vi "Untitled 1.vi"() -> ()   [LabVIEW 2023]
uses:
  Control Timer.ctl
panel:
  out "Mixing":bool
  out "Boiling milk":bool
  out "Adding Milk":bool
  out "Boiling":bool
  out "Adding Coffee":bool
  out "Adding Water":bool
  in  "WHITE COFFEE":bool
  in  "CAPUCCINO":bool
  in  "ESPRESSO LONG":bool
  in  "ESPRESSO SHORT":bool
  in  "STOP":bool
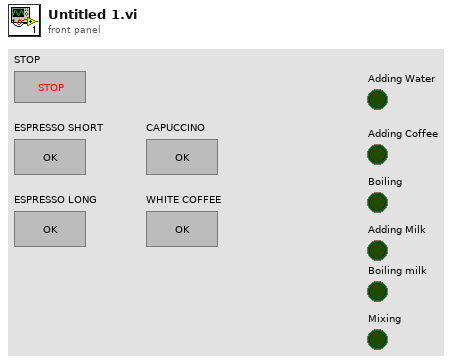
[diagram p1: front panel]
types:
  T1 = typedef "Control Timer.ctl" = enum16{"Timecheck", "Reset"}
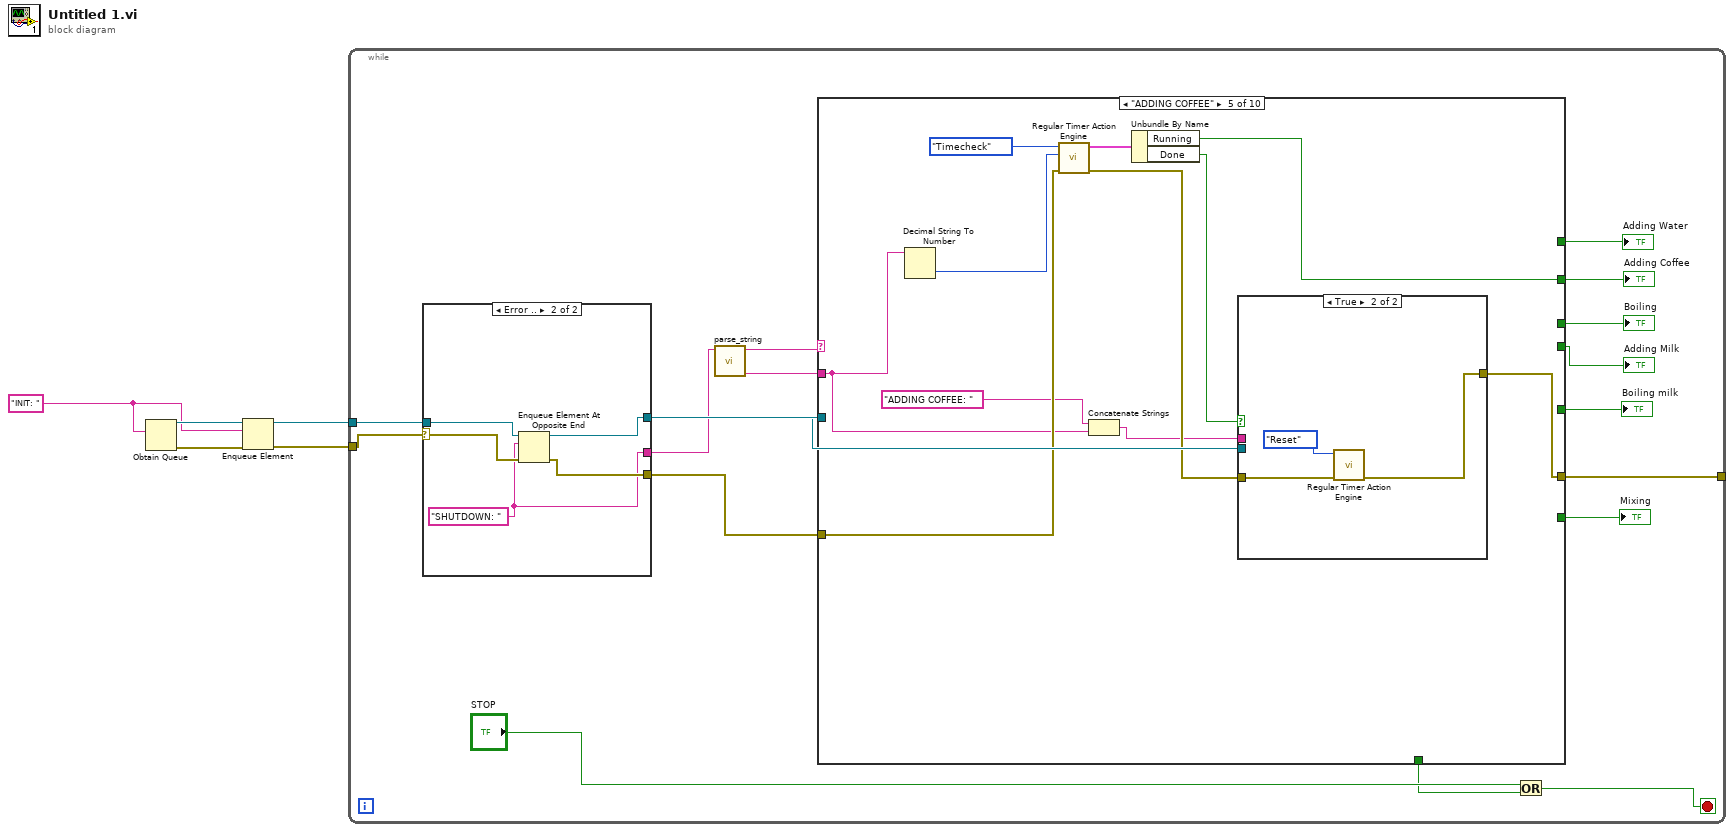
[diagram p0: block diagram]
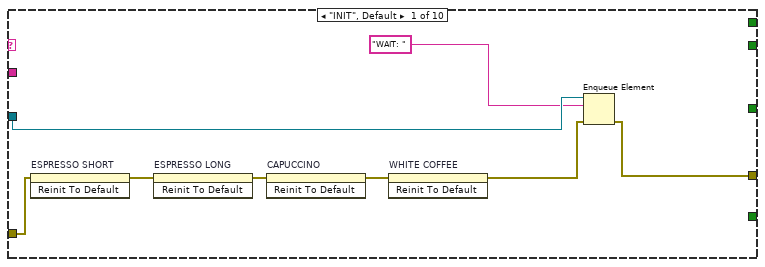
[diagram p2: hidden frame]
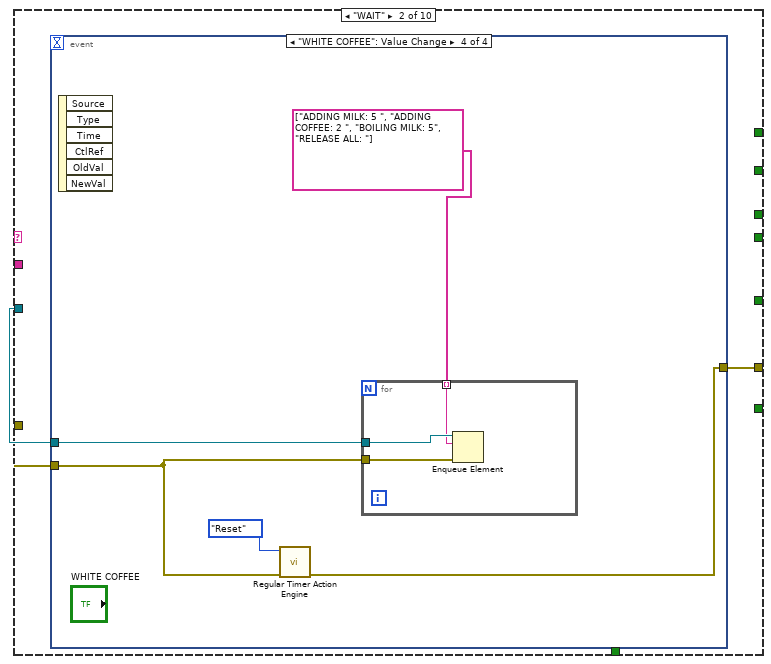
[diagram p3: hidden frame]
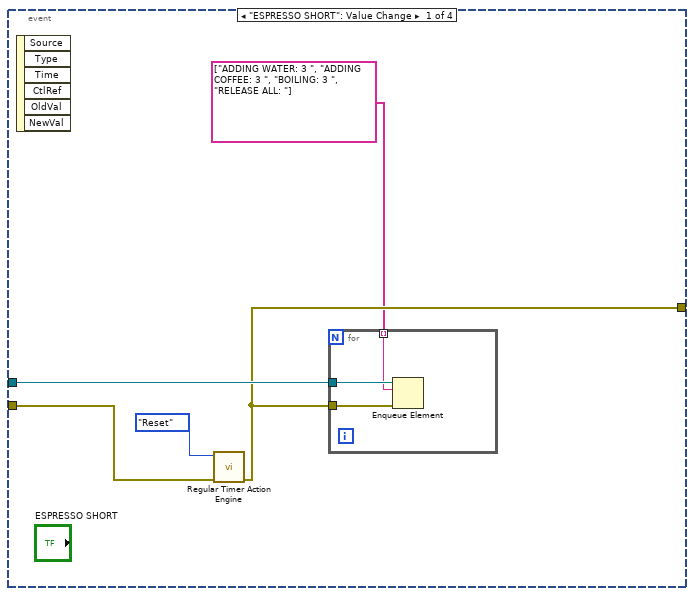
[diagram p4: hidden frame]
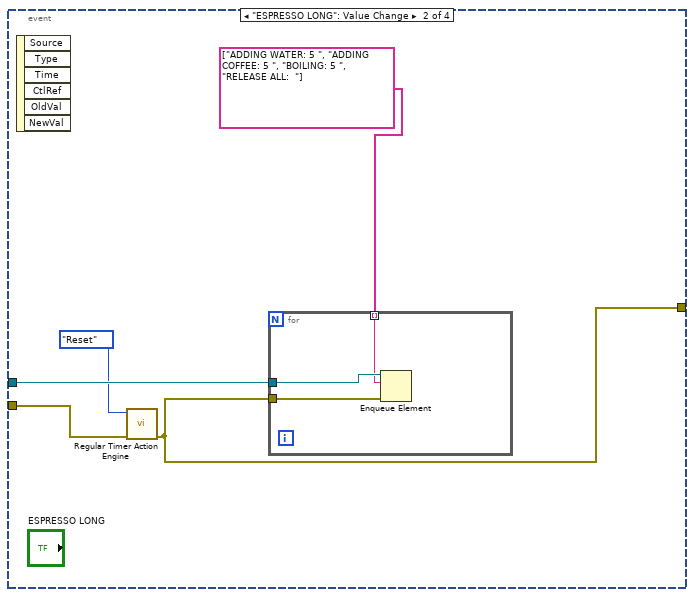
[diagram p5: hidden frame]
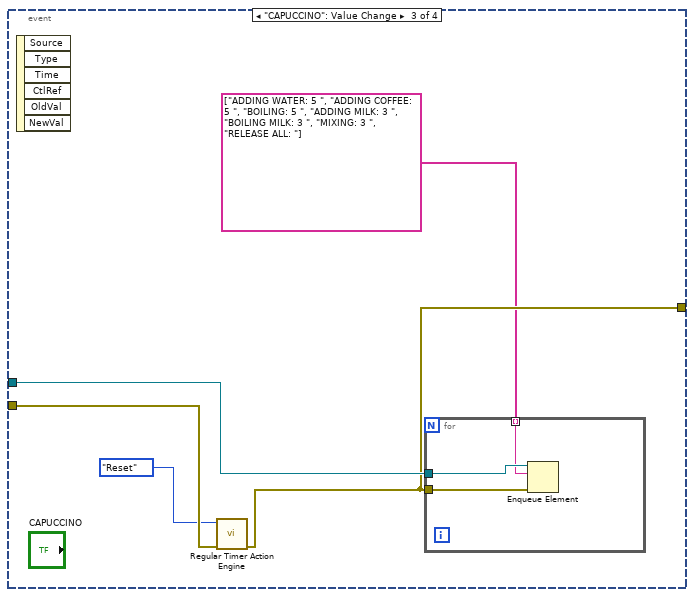
[diagram p6: hidden frame]
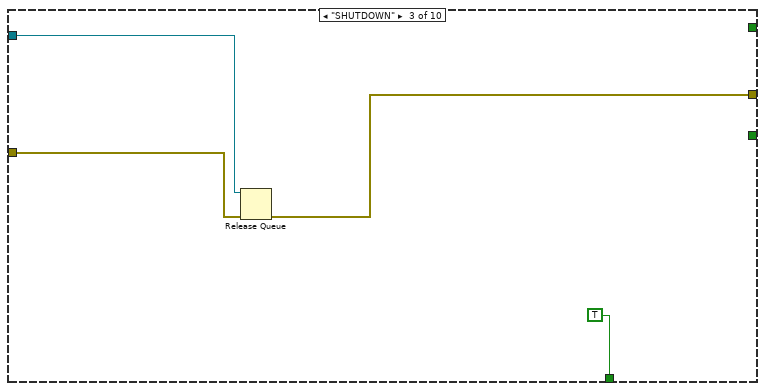
[diagram p7: hidden frame]
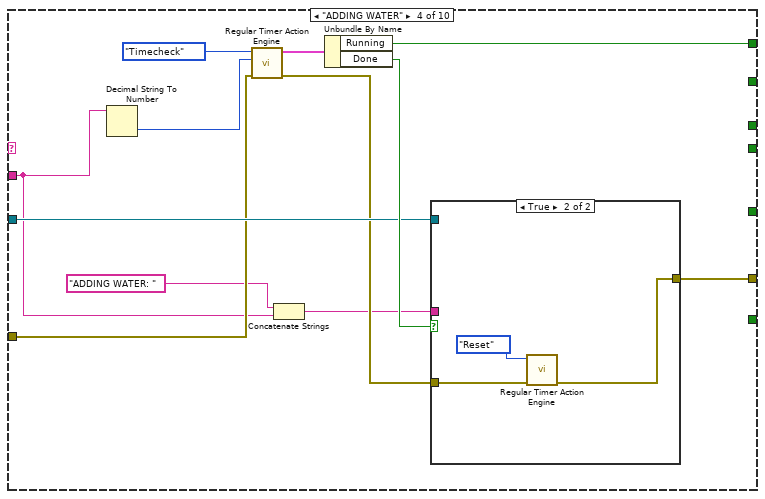
[diagram p8: hidden frame]
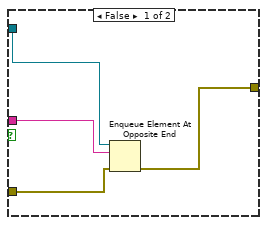
[diagram p9: hidden frame]
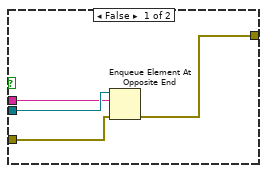
[diagram p10: hidden frame]
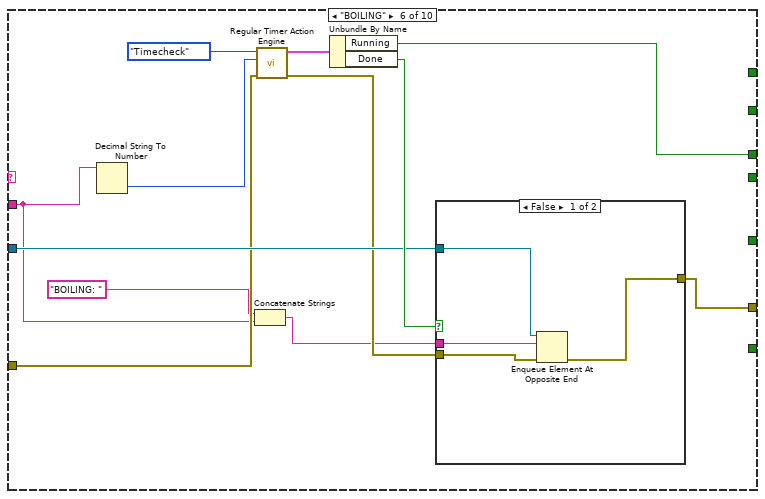
[diagram p11: hidden frame]
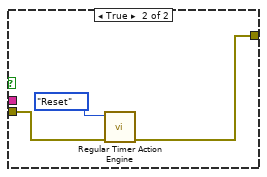
[diagram p12: hidden frame]
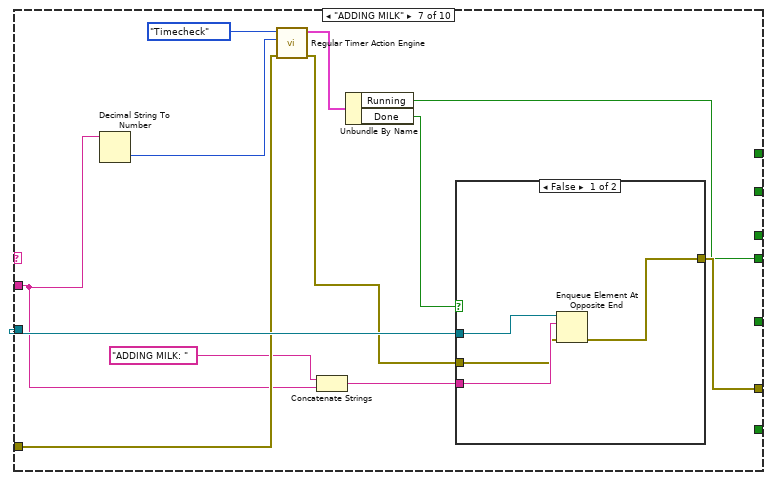
[diagram p13: hidden frame]
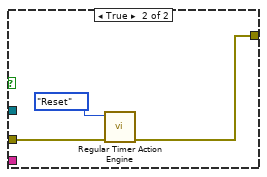
[diagram p14: hidden frame]
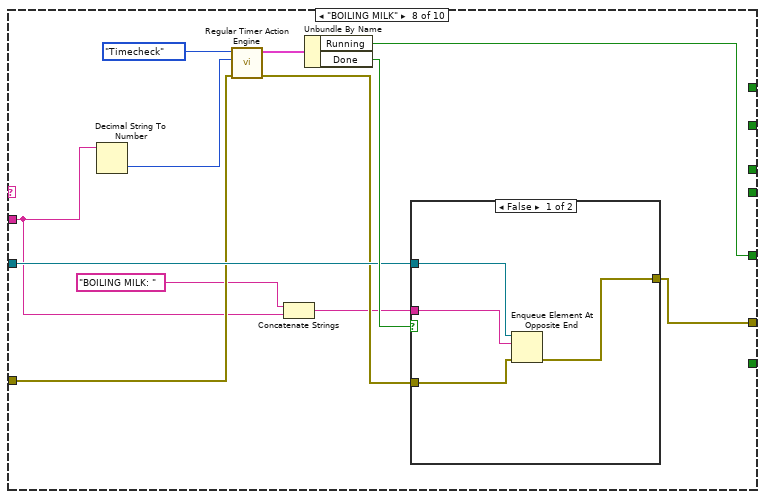
[diagram p15: hidden frame]
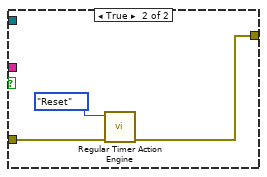
[diagram p16: hidden frame]
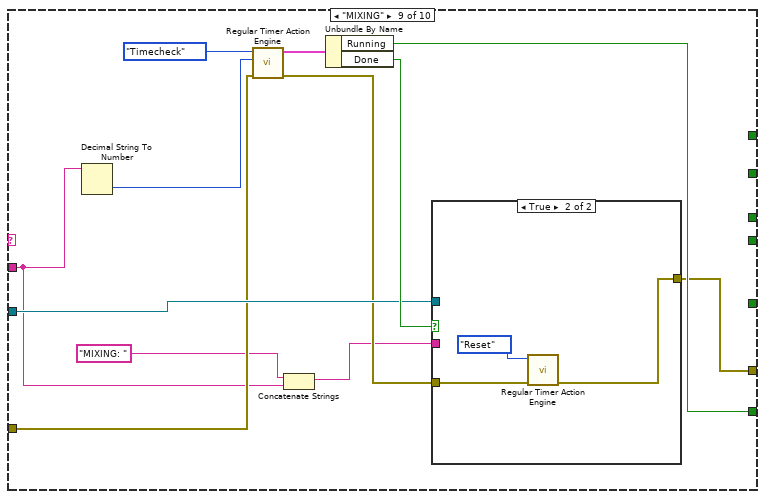
[diagram p17: hidden frame]
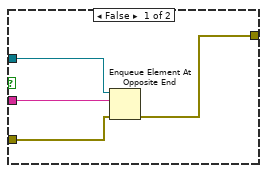
[diagram p18: hidden frame]
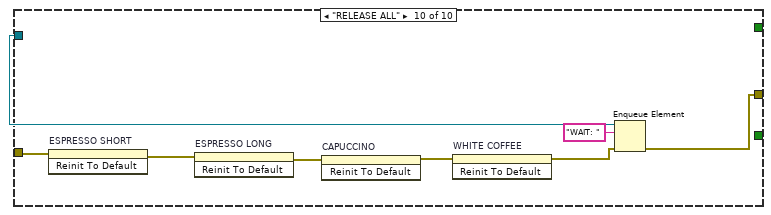
[diagram p19: hidden frame]
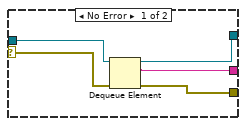
[diagram p20: hidden frame]
diagram:
  w1 = "INIT: "
  n1 = Obtain Queue(element data type=w1) -> (queue out=w5:refnum<queue>, error out=w4:errorcluster)  [unwired: 4 in, 1 out]
  n2 = Enqueue Element(queue=w5, element=w1, error in (no error)=w4) -> (queue out=w2:refnum<queue>, error out=w3:errorcluster)  [unwired: 1 in, 1 out]
  n3 = while {
    tunnel: w3 -> [w22]
    tunnel: w2 -> [w21]
    tunnel: [w18] -> _
    stop <- w9 stop-if-true
    n4 = case shown="Error .." w22 {
      selector: w22 -> [w196 w201]
      tunnel: w21 -> [w195 w199]
      tunnel: [w194 w198] -> w19
      tunnel: [w193 w200] -> w20
      tunnel: [w192 w197] -> w6
      frame No Error {
        n5 = Dequeue Element(queue=w195, error in (no error)=w196) -> (queue out=w194:refnum<queue>, element=w192:string, error out=w193:errorcluster)  [unwired: 1 in, 1 out]
      }
      frame Error {
        w197 = "SHUTDOWN: "
        n6 = Enqueue Element At Opposite End(queue=w199, element=w197, error in (no error)=w201) -> (queue out=w198:refnum<queue>, error out=w200:errorcluster)  [unwired: 1 in, 1 out]
      }
    }
    n7 = call "parse_string.vi"("Input"=w6) -> ("Argument"=w7:string, "State"=w8:string)  [unwired: 9 in]
    n8 = case shown="\"ADDING COFFEE\"" w8 {
      tunnel: w20 -> [w24 w32 w69 w75 w94 w113 w132 w151 w169 w191]
      tunnel: w19 -> [w30 w33 w68 w76 w97 w116 w134 w154 w172 w186]
      tunnel: [w25 w31 w66 w77 w95 w114 w135 w152 w170 w185] -> w18
      tunnel: [_ _ _ w79 _ _ _ _ _ _] -> w17
      tunnel: [_ _ _ _ w96 _ _ _ _ _] -> w16
      tunnel: [_ _ _ _ _ w115 _ _ _ _] -> w15
      tunnel: [_ _ _ _ _ _ w133 _ _ _] -> w14
      tunnel: [_ _ _ _ _ _ _ w153 _ _] -> w13
      tunnel: [_ _ _ _ _ _ _ _ w171 _] -> w12
      tunnel: [_ _ TRUE _ _ _ _ _ _ _] -> w10
      tunnel: w7 -> [_ _ _ w70 w89 w108 w127 w146 w165 _]
      frame "INIT", Default {
        n9 = invoke on="ESPRESSO SHORT" class="Bool" method="Reinit To Default"(error in=w24) -> (error out=w29:errorcluster)  [unwired: 2 in, 2 out]
        n10 = invoke on="ESPRESSO LONG" class="Bool" method="Reinit To Default"(error in=w29) -> (error out=w28:errorcluster)  [unwired: 2 in, 2 out]
        n11 = invoke on="CAPUCCINO" class="Bool" method="Reinit To Default"(error in=w28) -> (error out=w27:errorcluster)  [unwired: 2 in, 2 out]
        n12 = invoke on="WHITE COFFEE" class="Bool" method="Reinit To Default"(error in=w27) -> (error out=w26:errorcluster)  [unwired: 2 in, 2 out]
        n13 = Enqueue Element(queue=w30, element="WAIT: ", error in (no error)=w26) -> (error out=w25:errorcluster)  [unwired: 1 in, 2 out]
      }
      frame "WAIT" {
        n14 = event shown="[3] \"WHITE COFFEE\": Value Change" {
          selector: _ -> [_ _ _ _]
          dyn-events: _ -> [_ _ _ _]
          timeout: _ -> [_ _ _ _]
          tunnel: w33 -> [w38 w46 w54 w62]
          tunnel: w32 -> [w36 w44 w53 w59]
          tunnel: [w35 w43 w51 w60] -> w31
          event "ESPRESSO SHORT": Value Change {
            n15 = event-data() -> ()  [unwired: 1 in, 6 out]
            n16 = call "Regular Timer Action Engine.vi"("Enum"=Control_Timer."Reset", "error in"=w36) -> ("error out"=w35:errorcluster)  [unwired: 7 in, 1 out]
            n17 = for {
              tunnel: w38 -> [w41]
              tunnel: w35 -> [w40]
              tunnel: string[] ["ADDING WATER: 3 ", "ADDING COFFEE: 3 ", "BOILING: 3 ", "RELEASE ALL: "] -> [w39] mode=indexing
              n18 = Enqueue Element(queue=w41, element=w39, error in (no error)=w40) -> ()  [unwired: 1 in, 3 out]
            }
          }
          event "ESPRESSO LONG": Value Change {
            n19 = event-data() -> ()  [unwired: 1 in, 6 out]
            n20 = call "Regular Timer Action Engine.vi"("Enum"=Control_Timer."Reset", "error in"=w44) -> ("error out"=w43:errorcluster)  [unwired: 7 in, 1 out]
            n21 = for {
              tunnel: w46 -> [w49]
              tunnel: w43 -> [w48]
              tunnel: string[] ["ADDING WATER: 5 ", "ADDING COFFEE: 5 ", "BOILING: 5 ", "RELEASE ALL:  "] -> [w47] mode=indexing
              n22 = Enqueue Element(queue=w49, element=w47, error in (no error)=w48) -> ()  [unwired: 1 in, 3 out]
            }
          }
          event "CAPUCCINO": Value Change {
            n23 = event-data() -> ()  [unwired: 1 in, 6 out]
            n24 = call "Regular Timer Action Engine.vi"("Enum"=Control_Timer."Reset", "error in"=w53) -> ("error out"=w51:errorcluster)  [unwired: 7 in, 1 out]
            n25 = for {
              tunnel: w54 -> [w57]
              tunnel: w51 -> [w56]
              tunnel: string[] ["ADDING WATER: 5 ", "ADDING COFFEE: 5 ", "BOILING: 5 ", "ADDING MILK: 3 ", "BOILING MILK: 3 ", "MIXING: 3 ", "RELEASE ALL: "] -> [w55] mode=indexing
              n26 = Enqueue Element(queue=w57, element=w55, error in (no error)=w56) -> ()  [unwired: 1 in, 3 out]
            }
          }
          event "WHITE COFFEE": Value Change {
            n27 = event-data() -> ()  [unwired: 1 in, 6 out]
            n28 = call "Regular Timer Action Engine.vi"("Enum"=Control_Timer."Reset", "error in"=w59) -> ("error out"=w60:errorcluster)  [unwired: 7 in, 1 out]
            n29 = for {
              tunnel: w62 -> [w65]
              tunnel: w59 -> [w64]
              tunnel: string[] ["ADDING MILK: 5 ", "ADDING COFFEE: 2 ", "BOILING MILK: 5", "RELEASE ALL: "] -> [w63] mode=indexing
              n30 = Enqueue Element(queue=w65, element=w63, error in (no error)=w64) -> ()  [unwired: 1 in, 3 out]
            }
          }
        }
      }
      frame "SHUTDOWN" {
        n31 = Release Queue(queue=w68, error in (no error)=w69) -> (error out=w66:errorcluster)  [unwired: 1 in, 2 out]
      }
      frame "ADDING WATER" {
        n32 = Decimal String To Number(string=w70) -> (number=w73:i32)  [unwired: 2 in, 1 out]
        n33 = call "Regular Timer Action Engine.vi"("Enum"=Control_Timer."Timecheck", "Time Target"=w73, "error in"=w75) -> ("Status"=w80:cluster{"Running":bool, "Done":bool}, "error out"=w74:errorcluster)  [unwired: 6 in]
        n34 = Concatenate Strings("ADDING WATER: ", w70) -> (w71:string)
        n35 = Unbundle By Name(w80) -> ("Running"=w79:bool, "Done"=w78:bool)
        n36 = case shown="True" w78 {
          tunnel: [w84 w87] -> w77
          tunnel: w76 -> [w85 _]
          tunnel: w74 -> [w83 w86]
          tunnel: w71 -> [w82 _]
          frame False {
            n37 = Enqueue Element At Opposite End(queue=w85, element=w82, error in (no error)=w83) -> (error out=w84:errorcluster)  [unwired: 1 in, 2 out]
          }
          frame True {
            n38 = call "Regular Timer Action Engine.vi"("Enum"=Control_Timer."Reset", "error in"=w86) -> ("error out"=w87:errorcluster)  [unwired: 7 in, 1 out]
          }
        }
      }
      frame "ADDING COFFEE" {
        n39 = Decimal String To Number(string=w89) -> (number=w92:i32)  [unwired: 2 in, 1 out]
        n40 = call "Regular Timer Action Engine.vi"("Enum"=Control_Timer."Timecheck", "Time Target"=w92, "error in"=w94) -> ("Status"=w99:cluster{"Running":bool, "Done":bool}, "error out"=w93:errorcluster)  [unwired: 6 in]
        n41 = Concatenate Strings("ADDING COFFEE: ", w89) -> (w90:string)
        n42 = Unbundle By Name(w99) -> ("Running"=w96:bool, "Done"=w98:bool)
        n43 = case shown="True" w98 {
          tunnel: [w104 w106] -> w95
          tunnel: w97 -> [w103 _]
          tunnel: w93 -> [w101 w105]
          tunnel: w90 -> [w102 _]
          frame False {
            n44 = Enqueue Element At Opposite End(queue=w103, element=w102, error in (no error)=w101) -> (error out=w104:errorcluster)  [unwired: 1 in, 2 out]
          }
          frame True {
            n45 = call "Regular Timer Action Engine.vi"("Enum"=Control_Timer."Reset", "error in"=w105) -> ("error out"=w106:errorcluster)  [unwired: 7 in, 1 out]
          }
        }
      }
      frame "BOILING" {
        n46 = Decimal String To Number(string=w108) -> (number=w111:i32)  [unwired: 2 in, 1 out]
        n47 = Concatenate Strings("BOILING: ", w108) -> (w109:string)
        n48 = call "Regular Timer Action Engine.vi"("Enum"=Control_Timer."Timecheck", "Time Target"=w111, "error in"=w113) -> ("Status"=w118:cluster{"Running":bool, "Done":bool}, "error out"=w112:errorcluster)  [unwired: 6 in]
        n49 = Unbundle By Name(w118) -> ("Running"=w115:bool, "Done"=w117:bool)
        n50 = case shown="False" w117 {
          tunnel: [w123 w125] -> w114
          tunnel: w112 -> [w122 w124]
          tunnel: w116 -> [w121 _]
          tunnel: w109 -> [w120 _]
          frame False {
            n51 = Enqueue Element At Opposite End(queue=w121, element=w120, error in (no error)=w122) -> (error out=w123:errorcluster)  [unwired: 1 in, 2 out]
          }
          frame True {
            n52 = call "Regular Timer Action Engine.vi"("Enum"=Control_Timer."Reset", "error in"=w124) -> ("error out"=w125:errorcluster)  [unwired: 7 in, 1 out]
          }
        }
      }
      frame "ADDING MILK" {
        n53 = Decimal String To Number(string=w127) -> (number=w130:i32)  [unwired: 2 in, 1 out]
        n54 = call "Regular Timer Action Engine.vi"("Enum"=Control_Timer."Timecheck", "Time Target"=w130, "error in"=w132) -> ("Status"=w137:cluster{"Running":bool, "Done":bool}, "error out"=w131:errorcluster)  [unwired: 6 in]
        n55 = Concatenate Strings("ADDING MILK: ", w127) -> (w128:string)
        n56 = Unbundle By Name(w137) -> ("Running"=w133:bool, "Done"=w136:bool)
        n57 = case shown="False" w136 {
          tunnel: [w142 w144] -> w135
          tunnel: w134 -> [w141 _]
          tunnel: w131 -> [w139 w143]
          tunnel: w128 -> [w140 _]
          frame False {
            n58 = Enqueue Element At Opposite End(queue=w141, element=w140, error in (no error)=w139) -> (error out=w142:errorcluster)  [unwired: 1 in, 2 out]
          }
          frame True {
            n59 = call "Regular Timer Action Engine.vi"("Enum"=Control_Timer."Reset", "error in"=w143) -> ("error out"=w144:errorcluster)  [unwired: 7 in, 1 out]
          }
        }
      }
      frame "BOILING MILK" {
        n60 = Decimal String To Number(string=w146) -> (number=w149:i32)  [unwired: 2 in, 1 out]
        n61 = call "Regular Timer Action Engine.vi"("Enum"=Control_Timer."Timecheck", "Time Target"=w149, "error in"=w151) -> ("Status"=w156:cluster{"Running":bool, "Done":bool}, "error out"=w150:errorcluster)  [unwired: 6 in]
        n62 = Concatenate Strings("BOILING MILK: ", w146) -> (w147:string)
        n63 = Unbundle By Name(w156) -> ("Running"=w153:bool, "Done"=w155:bool)
        n64 = case shown="False" w155 {
          tunnel: [w161 w163] -> w152
          tunnel: w154 -> [w160 _]
          tunnel: w150 -> [w158 w162]
          tunnel: w147 -> [w159 _]
          frame False {
            n65 = Enqueue Element At Opposite End(queue=w160, element=w159, error in (no error)=w158) -> (error out=w161:errorcluster)  [unwired: 1 in, 2 out]
          }
          frame True {
            n66 = call "Regular Timer Action Engine.vi"("Enum"=Control_Timer."Reset", "error in"=w162) -> ("error out"=w163:errorcluster)  [unwired: 7 in, 1 out]
          }
        }
      }
      frame "MIXING" {
        n67 = Decimal String To Number(string=w165) -> (number=w175:i32)  [unwired: 2 in, 1 out]
        n68 = call "Regular Timer Action Engine.vi"("Enum"=Control_Timer."Timecheck", "Time Target"=w175, "error in"=w169) -> ("Status"=w174:cluster{"Running":bool, "Done":bool}, "error out"=w168:errorcluster)  [unwired: 6 in]
        n69 = Concatenate Strings("MIXING: ", w165) -> (w166:string)
        n70 = Unbundle By Name(w174) -> ("Running"=w171:bool, "Done"=w173:bool)
        n71 = case shown="True" w173 {
          tunnel: [w180 w182] -> w170
          tunnel: w172 -> [w179 _]
          tunnel: w168 -> [w178 w181]
          tunnel: w166 -> [w177 _]
          frame False {
            n72 = Enqueue Element At Opposite End(queue=w179, element=w177, error in (no error)=w178) -> (error out=w180:errorcluster)  [unwired: 1 in, 2 out]
          }
          frame True {
            n73 = call "Regular Timer Action Engine.vi"("Enum"=Control_Timer."Reset", "error in"=w181) -> ("error out"=w182:errorcluster)  [unwired: 7 in, 1 out]
          }
        }
      }
      frame "RELEASE ALL" {
        n74 = invoke on="ESPRESSO SHORT" class="Bool" method="Reinit To Default"(error in=w191) -> (error out=w190:errorcluster)  [unwired: 2 in, 2 out]
        n75 = invoke on="ESPRESSO LONG" class="Bool" method="Reinit To Default"(error in=w190) -> (error out=w189:errorcluster)  [unwired: 2 in, 2 out]
        n76 = invoke on="CAPUCCINO" class="Bool" method="Reinit To Default"(error in=w189) -> (error out=w188:errorcluster)  [unwired: 2 in, 2 out]
        n77 = invoke on="WHITE COFFEE" class="Bool" method="Reinit To Default"(error in=w188) -> (error out=w187:errorcluster)  [unwired: 2 in, 2 out]
        n78 = Enqueue Element(queue=w186, element="WAIT: ", error in (no error)=w187) -> (error out=w185:errorcluster)  [unwired: 1 in, 2 out]
      }
    }
    "Adding Water" <- w17
    "Adding Coffee" <- w16
    "Boiling" <- w15
    "Adding Milk" <- w14
    "Boiling milk" <- w13
    "Mixing" <- w12
    n79 = Or(x="STOP", y=w10) -> (x .or. y?=w9:bool)
  }
